vi "Direction.vi"(7 "RMS minimum\nvalues":T1, 8 "IRMS values":dbl[](array[numeric]), 9 "VRMS values":dbl[](array[numeric]), 10 "I array":waveform(sgl)[](array[waveform]), 11 "VL array":waveform(sgl)[](array[waveform])) -> (2 "Direction":enum16{"forward", "backward", "N/D"}(ring))   [LabVIEW 2016]
uses:
  <vilib>/addons/Electrical Power/Basic/Measurement/Power (N Channels).vi
  <vilib>/addons/Electrical Power/Basic/NI_EP_Basic.lvlib
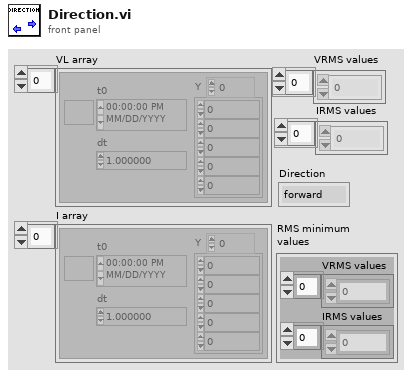
[diagram p1: front panel]
types:
  T1 = cluster{"VRMS values":dbl[], "IRMS values":dbl[]}
  T2 = typedef "NI_EP_Basic.lvlib/basic_Power Value.ctl" = cluster{"active power [W]":dbl, "apparent power [VA]":dbl, "reactive power [VAR]":dbl, "power factor":dbl}
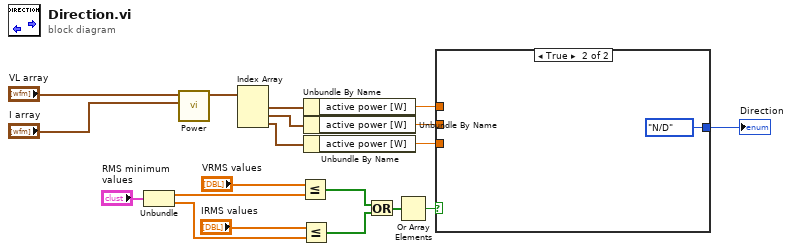
[diagram p0: block diagram]
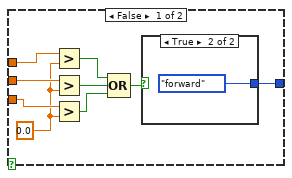
[diagram p2: hidden frame]
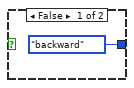
[diagram p3: hidden frame]
diagram:
  n1 = Unbundle("RMS minimum\nvalues") -> ("VRMS values"=w12:dbl[], "IRMS values"=w11:dbl[])
  n2 = call-poly <vilib>:"Power.vi"("current waveforms"="I array", "voltage waveforms"="VL array") -> ("power values"=w19:T2[])  [unwired: 8 in, 1 out]
  n3 = Index Array(array=w19) -> (element #1=w18:T2, element #2=w17:T2, element #3=w16:T2)  [unwired: 3 in]
  n4 = Less Or Equal?(x="VRMS values", y=w12) -> (x <= y?=w10:bool[])
  n5 = Less Or Equal?(x="IRMS values", y=w11) -> (x <= y?=w9:bool[])
  n6 = Unbundle By Name(w18) -> ("active power [W]"=w6:dbl)
  n7 = Unbundle By Name(w17) -> ("active power [W]"=w5:dbl)
  n8 = Unbundle By Name(w16) -> ("active power [W]"=w4:dbl)
  n9 = Or(x=w10, y=w9) -> (x .or. y?=w8:bool[])
  n10 = Or Array Elements(Boolean array=w8) -> (logical OR=w7:bool)
  n11 = case shown="True" w7 {
    tunnel: w6 -> [w28 _]
    tunnel: w5 -> [w27 _]
    tunnel: w4 -> [w26 _]
    tunnel: [w20 enum16{"forward", "backward", "N/D"}."N/D"] -> w3
    frame False {
      w25 = 0.0 ("y")
      n12 = Greater?(x=w28, y=w25) -> (0:w24:bool)
      n13 = Greater?(x=w27, y=w25) -> (0:w23:bool)
      n14 = Greater?(x=w26, y=w25) -> (0:w22:bool)
      n15 = Compound Arithmetic op=OR(w24, w23, w22) -> (w21:bool)
      n16 = case shown="True" w21 {
        tunnel: [enum16{"forward", "backward", "N/D"}."backward" enum16{"forward", "backward", "N/D"}."forward"] -> w20
        frame False {
        }
        frame True {
        }
      }
    }
    frame True {
    }
  }
  "Direction" <- w3
